vi "magboard_128_calibrate_nodes.vi"(11 "Sensor Input (mT)":dbl[][](array[numeric])) -> (3 "Sensor Output - Position (mm)":dbl[][](array[numeric]))   [LabVIEW 2018]
uses:
  FGVs/FGV States.ctl
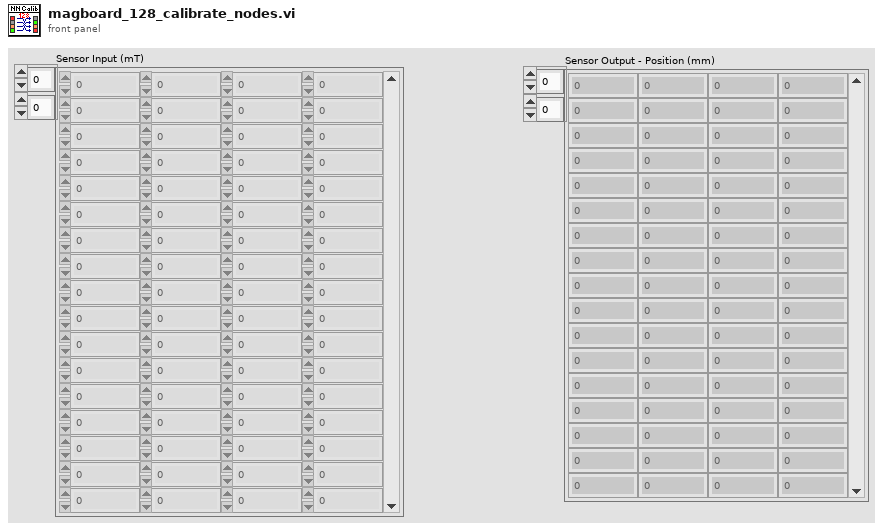
[diagram p1: front panel]
types:
  T1 = typedef "FGV States.ctl" = enum16{"Get", "Set", "Reset"}
  T2 = cluster{cluster{dbl[][], "Array":dbl[][]}, cluster{dbl[][], "Array":dbl[][]}, cluster{dbl[][], "Array":dbl[][]}, cluster{dbl[][], "Array":dbl[][]}}[]
  T3 = cluster{cluster{dbl[][], "Array":dbl[][]}, cluster{dbl[][], "Array":dbl[][]}, cluster{dbl[][], "Array":dbl[][]}, cluster{dbl[][], "Array":dbl[][]}}
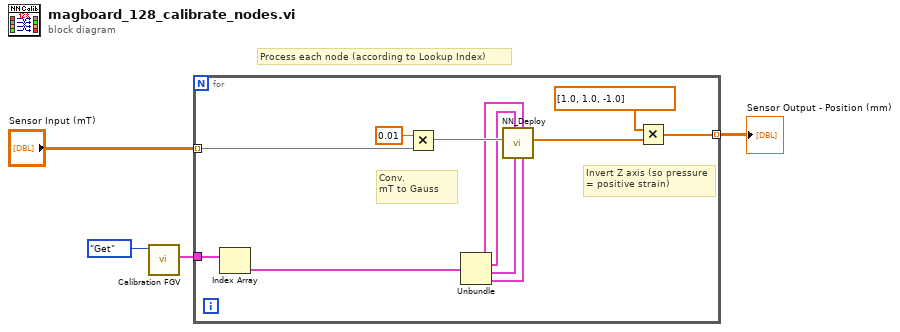
[diagram p0: block diagram]
diagram:
  # "Process each node (according to Lookup Index)"
  n1 = call "Calibration FGV.vi"("FGV States"=FGV_States."Get") -> ("Calib in 2"=w3:T2)  [unwired: 10 in]
  n2 = for {
    tunnel: w3 -> [w10]
    tunnel: [w6] -> w2 mode=indexing
    tunnel: "Sensor Input (mT)" -> [w8] mode=indexing
    # "Invert Z axis (so pressure\n= positive strain)"
    # "Conv. \nmT to Gauss"
    n3 = Index Array(array=w10) -> (element=w9:T3)  [unwired: 1 in]
    n4 = Multiply(x=0.01, y=w8) -> (x*y=w15:dbl[])
    n5 = Unbundle(w9) -> (w14:cluster{dbl[][], "Array":dbl[][]}, w13:cluster{dbl[][], "Array":dbl[][]}, w12:cluster{dbl[][], "Array":dbl[][]}, w11:cluster{dbl[][], "Array":dbl[][]})
    n6 = call "NN_Deploy.vi"("Output Layer"=w11, "Input Layer"=w14, "Layer 2"=w12, "Layer 1"=w13, "Input"=w15) -> ("Output"=w7:dbl[])  [unwired: 6 in]
    n7 = Multiply(x=dbl[] [1.0, 1.0, -1.0], y=w7) -> (x*y=w6:dbl[])
  }
  "Sensor Output - Position (mm)" <- w2
